vi "Holding Register Get Data Type.vi"(8 "error in (no error)":errorcluster, 11 "Item Ref in":T2 format="%.0x") -> (0 "error out":errorcluster, 2 "Data Type":T1, 3 "Item Ref out":T2 format="%.0x")   [LabVIEW 2015, in "Modbus Master System Explorer.lvlib"]
uses:
  Modbus Master System Explorer.lvlib
  <vilib>/NI Veristand/Custom Device API/Custom Device Item Ref.ctl
  Shared/Controls/Data Model/DataType.ctl
  Shared/Constants.vi
  <vilib>/NI Veristand/Custom Device API/Get Item Property (U16).vi
  <vilib>/NI VeriStand/Custom Device API/Custom Device API.lvlib
  Shared/Modbus Master Shared.lvlib
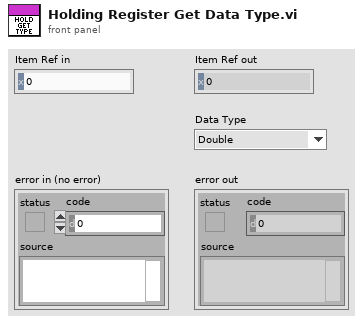
[diagram p1: front panel]
types:
  T1 = typedef "Modbus Master Shared.lvlib/DataType.ctl" = enum16{"Double", "Single", "I64", "I32", "I16", "I8", "U64", "U32", "U16", "U8", "Boolean"}
  T2 = typedef "Custom Device API.lvlib/Custom Device Item Ref.ctl" = u64
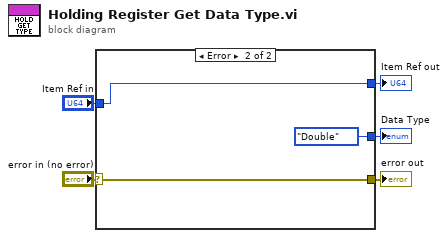
[diagram p0: block diagram]
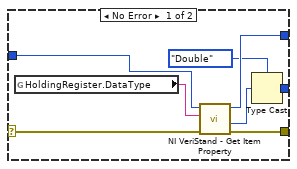
[diagram p2: hidden frame]
diagram:
  n1 = case shown="Error" "error in (no error)" {
    selector: "error in (no error)" -> [w12 w15]
    tunnel: "Item Ref in" -> [w11 w16]
    tunnel: [w10 w15] -> w3
    tunnel: [w9 w16] -> w2
    tunnel: [w6 DataType."Double" ("DataType")] -> w1
    frame No Error {
      n2 = global read "Constants.vi" "HoldingRegister.DataType"() -> (w13:string)
      n3 = call-poly <vilib>:"NI VeriStand - Get Item Property.vi"("error in (no error)"=w12, "Property Name"=w13, "Item Ref in"=w11) -> ("error out"=w10:errorcluster, "Value"=w7:u16, "Item Ref out"=w9:T2)  [unwired: 5 in, 1 out]
      n4 = Type Cast(type=DataType."Double" ("DataType"), x=w7) -> (*(type *) &x=w6:T1)
    }
    frame Error {
    }
  }
  "error out" <- w3
  "Item Ref out" <- w2
  "Data Type" <- w1
